vi "Game Data to Boolean Array.vi"(1 "Game Data":string) -> (0 "Is Right?":bool[](array[boolean]))   [LabVIEW 2017]
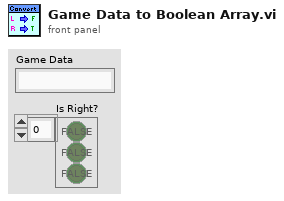
[diagram p1: front panel]
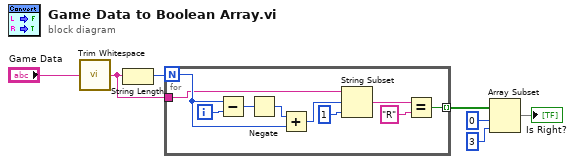
[diagram p0: block diagram]
diagram:
  n1 = call <vilib>:"Trim Whitespace.vi"("string"="Game Data") -> ("trimmed string"=w5:string)  [unwired: 1 in]
  n2 = String Length(string=w5) -> (length=w7:i32)
  n3 = for {
    N: w7 -> [w13]
    tunnel: w5 -> [w11]
    tunnel: [w8] -> w4 mode=indexing
    i -> [w12]
    n4 = Subtract(x=w13, y=w12) -> (x-y=w15:i32)
    n5 = Negate(x=w15) -> (-x=w16:i32)
    n6 = Add(x=w16, y=w13) -> (x+y=w17:i32)
    n7 = String Subset(string=w11, offset (0)=w17, length (rest)=1 ("length (rest)")) -> (substring=w10:string)
    n8 = Equal?(x=w10, y="R") -> (x = y?=w8:bool)
  }
  n9 = Array Subset(array=w4, index=0, length=3) -> (→"Is Right?":bool[])
